vi "Ctor.vi"(8 "error in (no error)":errorcluster, 11 "TCPConfigPanel in":refnum<class "TCPConfigPanel.lvclass">) -> (0 "error out":errorcluster, 3 "TCPConfigPanel out":refnum<class "TCPConfigPanel.lvclass">)   [LabVIEW 2020, in "LV-Term.lvlib" / "TCPConfigPanel.lvclass"]
uses:
  TCPConfigPanel.lvclass
  TCPConfigPanel.lvclass/TCPConfigPanel.ctl
  Ref Data.ctl
  <vilib>/IlluminatedG/IG OOPanel/OOPanel/Panel/Panel.lvclass
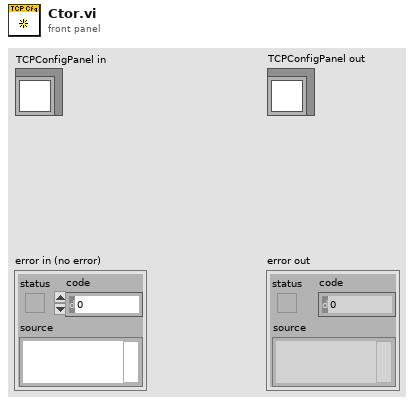
[diagram p1: front panel]
types:
  T1 = typedef "LV-Term.lvlib/TCPConfigPanel.lvclass/Ref Data.ctl" = cluster{"Host":string, "Port":u16}
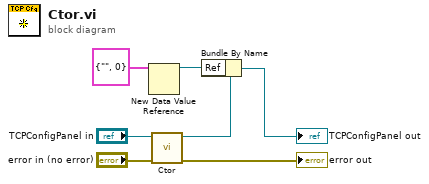
[diagram p0: block diagram]
diagram:
  n1 = New Data Value Reference(data value=T1 {"Host"="", "Port"=0} ("Ref Data")) -> (data value reference=w5:refnum<data-value>)  [unwired: 1 in, 1 out]
  n2 = call-parent "Ctor.vi"("error in (no error)"="error in (no error)", "Panel in"="TCPConfigPanel in") -> ("error out"=→"error out":errorcluster, "Panel out"=w4:refnum<class "TCPConfigPanel.lvclass">)  [unwired: 8 in]
  n3 = Bundle By Name(cluster=w4, "Ref"=w5) -> (→"TCPConfigPanel out":refnum<class "TCPConfigPanel.lvclass">)
